vi "Read Credentials.vi"(8 "error in (no error)":errorcluster, 11 "AWS Core in":refnum<class "NI_AWS_Core.lvclass">) -> (0 "error out":errorcluster, 2 "Credentials":T1, 3 "AWS Core out":refnum<class "NI_AWS_Core.lvclass">)   [LabVIEW 2015, in "NI_AWS_Core.lvclass"]
uses:
  NI_AWS_Core.lvclass
  AWS Credentials.ctl
  NI_AWS_Core.lvclass/NI_AWS_Core.ctl
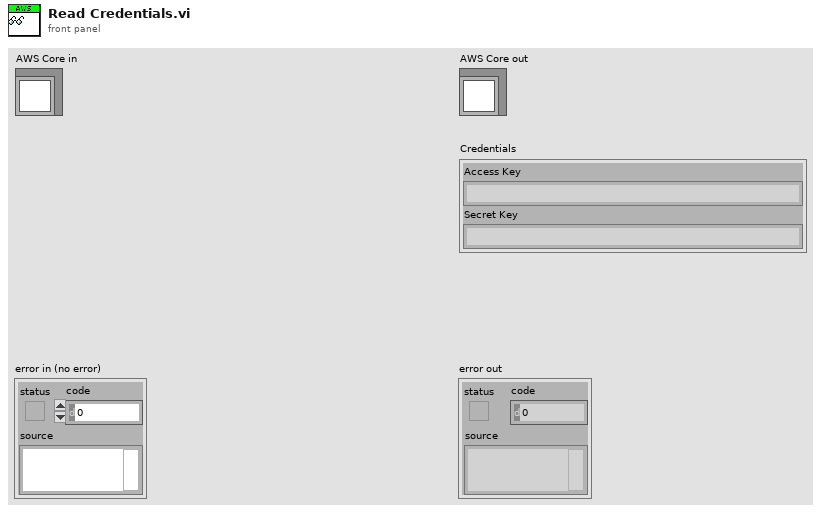
[diagram p1: front panel]
types:
  T1 = typedef "NI_AWS_Core.lvclass/AWS Credentials.ctl" = cluster{"Access Key":string, "Secret Key":string}
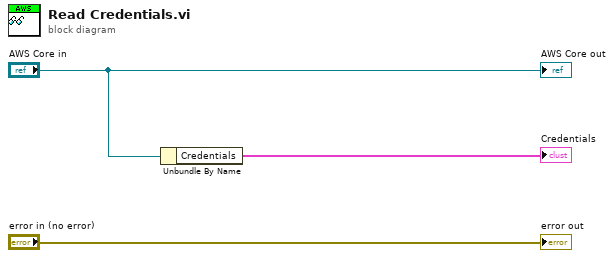
[diagram p0: block diagram]
diagram:
  n1 = Unbundle By Name("AWS Core in") -> ("Credentials"=→"Credentials":T1)
  "error out" <- "error in (no error)"
  "AWS Core out" <- "AWS Core in"
